vi "Read Design Request Key to Value.vi"(10 "Request Keys":T3, 11 "DesignRequest":T1) -> (3 "Value":string)   [LabVIEW 2012, in "Design Server.lvlib"]
uses:
  Design Server.lvlib
  RequestKeys.ctl
  Design Request.ctl
  Variable cluster.ctl
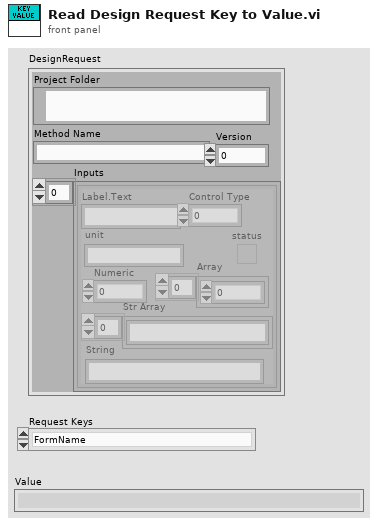
[diagram p1: front panel]
types:
  T1 = typedef "Design Server.lvlib/Design Request.ctl" = cluster{"Project Folder":path, "Method Name":string, "Inputs":T2, "Version":i32}
  T2 = typedef "Design Server.lvlib/Variable cluster.ctl" = cluster{"Label.Text":string, "Control Type":u32, "Numeric":dbl, "Array":dbl[], "status":bool, "Str Array":string[], "String":string, "unit":string}[]
  T3 = typedef "Design Server.lvlib/RequestKeys.ctl" = enum16{"FormName", "Name", "Email", "Organization", "Country", "ProjectTitle", "ProjectCity", "ProjectState", "ProjectNotes"}
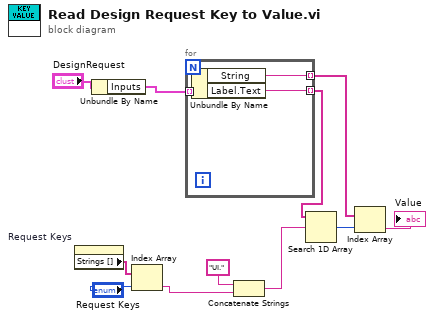
[diagram p0: block diagram]
diagram:
  n1 = property on="Request Keys" class="Enum (strict)"() -> ("Strings []"=w11:string[])  [unwired: 2 in, 2 out]
  n2 = Unbundle By Name("DesignRequest") -> ("Inputs"=w6:T2)
  n3 = Index Array(array=w11, index="Request Keys") -> (element=w3:string)
  n4 = for {
    tunnel: w6 -> [w14] mode=indexing
    tunnel: [w13] -> w4 mode=indexing
    tunnel: [w12] -> w5 mode=indexing
    n5 = Unbundle By Name(w14) -> ("String"=w12:string, "Label.Text"=w13:string)
  }
  n6 = Concatenate Strings("UI." ("string"), w3) -> (w1:string)
  n7 = Search 1D Array(1D array=w4, element=w1) -> (index of element=w9:i32)  [unwired: 1 in]
  n8 = Index Array(array=w5, index=w9) -> (element=→"Value":string)
